vi "MGI Find Rect Containing Point.vi"(1 "Mouse Position":cluster{"X":i16, "Y":i16}, 2 "Rectangle[]":T1(array[cluster])) -> (0 "First Rect(-1:none)":i32)   [LabVIEW 2016]
doc: "Return the index of the first rect containing the point, -1 if none.\n\nAuthored by David A. Moore\nsupport@mooregoodideas.com\nwww.mooregoodideas.com\n\nCopyright (c) 2010, Moore Good Ideas, Inc.\n\nAll rights reserved.\n\nRedistribution and use in source and binary forms, with or without modification, are permitted provided that the following conditions are met:\n\n * Redistributions of source code must retain the above copyright notice, this list of conditions and the following disclaimer.\n * Redistributions in binary form must reproduce the above copyright notice, this list of conditions and the following disclaimer in the documentation and/or other materials provided with the distribution.\n * Neither the name of Moore Good Ideas, Inc. nor the names of its contributors may be used to endorse or promote products derived from this software without specific prior written permission.\n\nTHIS SOFTWARE IS PROVIDED BY THE COPYRIGHT HOLDERS AND CONTRIBUTORS \"AS IS\" AND ANY EXPRESS OR IMPLIED WARRANTIES, INCLUDING, BUT NOT LIMITED TO, THE IMPLIED WARRANTIES OF MERCHANTABILITY AND FITNESS FOR A PARTICULAR PURPOSE ARE DISCLAIMED. IN NO EVENT SHALL THE COPYRIGHT OWNER OR CONTRIBUTORS BE LIABLE FOR ANY DIRECT, INDIRECT, INCIDENTAL, SPECIAL, EXEMPLARY, OR CONSEQUENTIAL DAMAGES (INCLUDING, BUT NOT LIMITED TO, PROCUREMENT OF SUBSTITUTE GOODS OR SERVICES; LOSS OF USE, DATA, OR PROFITS; OR BUSINESS INTERRUPTION) HOWEVER CAUSED AND ON ANY THEORY OF LIABILITY, WHETHER IN CONTRACT, STRICT LIABILITY, OR TORT (INCLUDING NEGLIGENCE OR OTHERWISE) ARISING IN ANY WAY OUT OF THE USE OF THIS SOFTWARE, EVEN IF ADVISED OF THE POSSIBILITY OF SUCH DAMAGE."
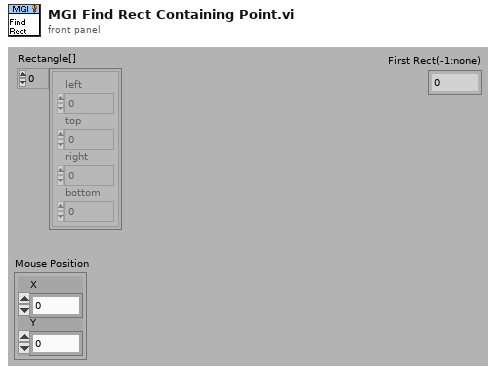
[diagram p1: front panel]
types:
  T1 = cluster{"left":i16, "top":i16, "right":i16, "bottom":i16}[]
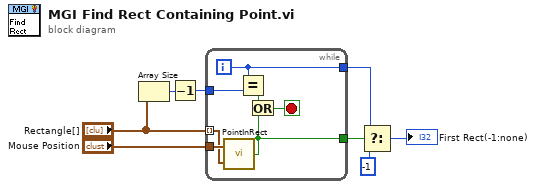
[diagram p0: block diagram]
diagram:
  n1 = Array Size(array="Rectangle[]") -> (size(s)=w6:i32)
  n2 = Decrement(x=w6) -> (x-1=w5:i32)
  n3 = while {
    tunnel: [w12] -> w3
    tunnel: [w11] -> w4
    tunnel: w5 -> [w15]
    tunnel: "Mouse Position" -> [w10]
    tunnel: "Rectangle[]" -> [w9] mode=indexing
    i -> [w12]
    stop <- w13 stop-if-true
    n4 = call <vilib>:"PointInRect.vi"("rect"=w9, "point"=w10) -> ("pt in rect"=w11:bool)
    n5 = Equal?(x=w12, y=w15) -> (x = y?=w14:bool)
    n6 = Or(x=w14, y=w11) -> (x .or. y?=w13:bool)
  }
  n7 = Select(t=w3, s=w4, f=-1) -> (s? t:f=→"First Rect(-1:none)":i32)
